vi "UpdateCamera.vi"(8 "error in (no error)":errorcluster, 11 "3D Scene in":refnum<class "3D Scene.lvclass">) -> (0 "error out":errorcluster, 3 "3D Scene out":refnum<class "3D Scene.lvclass">)   [LabVIEW 2015, in "3D Scene.lvclass"]
uses:
  3D Scene.lvclass
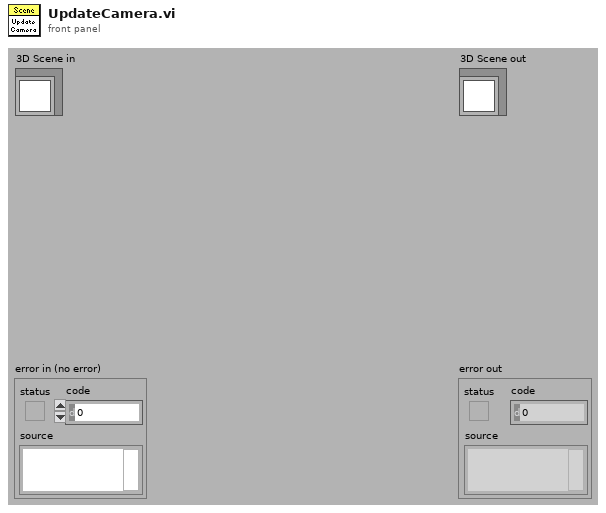
[diagram p1: front panel]
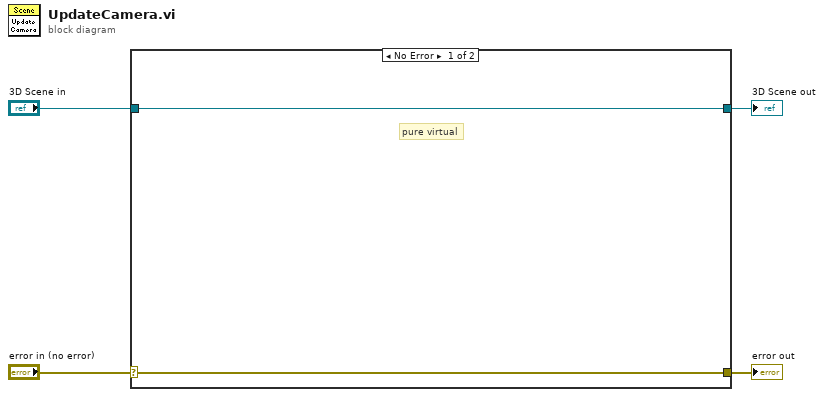
[diagram p0: block diagram]
diagram:
  n1 = case shown="No Error" "error in (no error)" {
    selector: "error in (no error)" -> [w5 w8]
    tunnel: [w5 w8] -> w3
    tunnel: [w6 w7] -> w1
    tunnel: "3D Scene in" -> [w6 w7]
    frame No Error {
      # "pure virtual"
    }
    frame Error {
    }
  }
  "error out" <- w3
  "3D Scene out" <- w1
